vi "Vision Research Phantom Series PhCon PhCineGet.vi"(0 "CN [in]":u32=1, 1 "Cine":i32, 2 "Sel":T1 items=["cgsVideoTone"=4097, "cgsName"=4098, "cgsVideoMarkIn"=4099, "cgsVideoMarkOut"=4100, "cgsIsRecorded"=4101, "cgsHqMode"=4102, "cgsBurstCount"=4103, "cgsBurstPeriod"=4104, "cgsLensDescription"=4105, "cgsLensAperature"=4106, "cgsLensFocalLength"=4107, "cgsShutterOff"=4108, "cgsTriggerTime"=4109, "cgsTrigTC"=4110, "cgsPbRate"=4111, "cgsTcRate"=4112, "cgsWb"=5100, "cgsBright"=5101, "cgsContrast"=5102, "cgsGamma"=5103, "cgsGammaR"=5109, "cgsGammaB"=5110, "cgsSaturation"=5104, "cgsHue"=5105, "cgsPedestalR"=5106, "cgsPedestalG"=5107, "cgsPedestalB"=5108, "cgsFlare"=5111, "cgsChroma"=5112, "cgsTone"=5113, "cgsUserMatrix"=5114, "cgsEnableMatrices"=5115], 5 "Error In (no error)":errorcluster) -> (14 "CN [out]":u32=1, 15 "pVal [out]":u64, 19 "Error Out":errorcluster)   [LabVIEW 2013, in "VRI.lvlib"]
doc: "PhCineGet\nHRESULT PhCineGet(UNIT CN, INT Cine, UINT Sel, PVOID pVal)\n\nParameters\nCN [in]\n Camera number.\nCine [in]\n Cine number.\nSel [in]\n Numerical selector identifying the parameter to be read.\npVal [out]\n Pointer where to store requested information.\n\nReturn Value\nThe function returns ERR_Ok in case of success or an error code, otherwise. To get extended error information call PhGetErrorMessage.\n\nRemarks\nThis function gets requested information for the specified camera cine. The cine is identified based on a cine number and the camera number it belongs to.\nCheck Appendix 3 for possible selector values.\nImportant! This is a low level function. Use it only if neither PhGetCineInfo nor PhGetCineParams can provide needed information. There is no interaction between this function and CINEHANDLE objects!\n\nRequired Header\nPhCon.h"
uses:
  VRI.lvlib
  _Type Defs/PhCon CGS.ctl
  Phantom DLLs/PhCon.dll
panel:
  # "For instructions on the use of this VI, press Ctrl+H to display the help window and move the mouse over the icon, controls, and indicators"
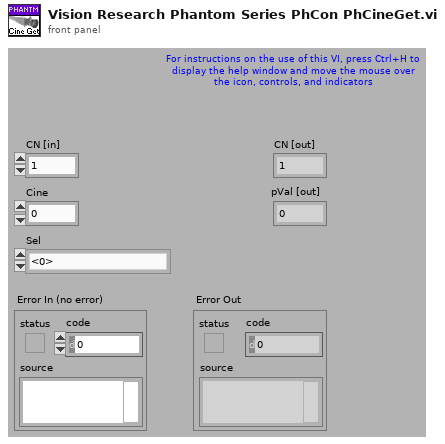
[diagram p1: front panel]
types:
  T1 = typedef "VRI.lvlib/PhCon CGS.ctl" = u16
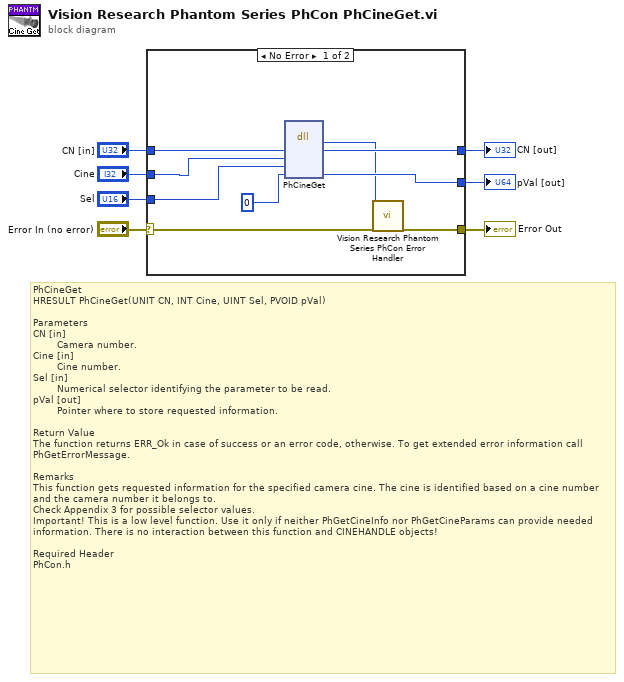
[diagram p0: block diagram]
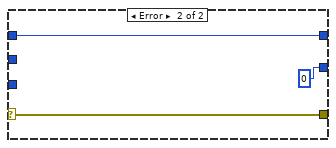
[diagram p2: hidden frame]
diagram:
  # "PhCineGet\nHRESULT PhCineGet(UNIT CN, INT Cine, UINT Sel, PVOID pVal)\n\nParameters\nCN [in]\n\t       Camera number.\nCine [in]\n\t       Cine number.\nSel [in]\n\t       Numerical selector identifying the parameter to be read.\npVal [out]\n\t       Pointer where to store requested information.\n\nReturn Value\nThe function returns ERR_Ok in case of success or an error code, otherwise. To get extended error information call PhGetErrorMessage.\n\nRemarks\nThis function gets requested information for the specified camera cine. The cine is identified based on a cine number and the camera number it belongs to.\nCheck Appendix 3 for possible selector values.\nImportant! This is a low level function. Use it only if neither PhGetCineInfo nor PhGetCineParams can provide needed information. There is no interaction between this function and CINEHANDLE objects!\n\nRequired Header\nPhCon.h"
  n1 = case shown="No Error" "Error In (no error)" {
    selector: "Error In (no error)" -> [w16 w19]
    tunnel: [w15 w19] -> w6
    tunnel: "CN [in]" -> [w14 w18]
    tunnel: [w13 w18] -> w4
    tunnel: "Sel" -> [w12 _]
    tunnel: [w11 u64 0 ("pVal")] -> w2
    tunnel: "Cine" -> [w10 _]
    frame No Error {
      n2 = dll-call lib="C:/Projects/SDK/32-bit/Vision Research Phantom Series Labview Driver/Phantom DLLs/PhCon.dll" fn="PhCineGet"("CN"=w14, "Cine"=w10, "Sel"=w12, "pVal"=u64 0) -> ("HRESULT"=w9:i32, "CN"=w13:u32, "pVal"=w11:u64)  [unwired: 4 in, 3 out]
      n3 = call "Vision Research Phantom Series PhCon Error Handler.vi"("ErrNo"=w9, "Error In (no error)"=w16) -> ("Error Out"=w15:errorcluster)  [unwired: 17 out]
    }
    frame Error {
    }
  }
  "Error Out" <- w6
  "CN [out]" <- w4
  "pVal [out]" <- w2
